vi "Sequence length convert.vi"(4 "Sequence":u8[](array[numeric])) -> (1 "Sequence Length":u8[](array[numeric]))   [LabVIEW 2017]
doc: "This VI is used to calculate and format the sequence length for a given sequence in a PDU. The output is a byte array containing the sequence length of the sequence passed in as input. The sequence length is calculated as per the SNMP specification."
panel:
  out "size(s)":i32
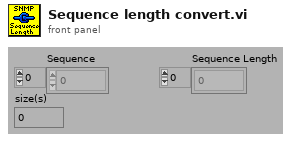
[diagram p1: front panel]
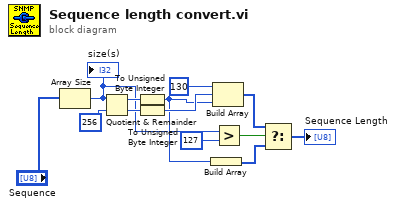
[diagram p0: block diagram]
diagram:
  n1 = Array Size(array="Sequence") -> (size(s)=w2:i32)
  "size(s)" <- w2
  n2 = Quotient & Remainder(x=w2, y=256) -> (x-y*floor(x/y)=w3:i32, floor(x/y)=w4:i32)
  n3 = To Unsigned Byte Integer(number=w3) -> (unsigned 8bit integer=w5:u8)
  n4 = To Unsigned Byte Integer(number=w4) -> (unsigned 8bit integer=w10:u8)
  n5 = Build Array(w5) -> (w6:u8[])
  n6 = Build Array(u8 130, w10, w5) -> (w8:u8[])
  n7 = Greater?(x=w2, y=127) -> (0:w9:bool)
  n8 = Select(t=w8, s=w9, f=w6) -> (s? t:f=→"Sequence Length":u8[])
